vi "Stop Core.vi"(10 "final error code":i32 caption="最终错误代码", 11 "DAQ in":refnum<class "DAQ.lvclass"> caption="操作者输入") -> (3 "DAQ out":refnum<class "DAQ.lvclass"> caption="操作者输出")   [LabVIEW 2017, in "DAQ.lvlib" / "DAQ.lvclass"]
doc: "(<B>Filename</B>: Actor Framework.lvlib:Actor.lvclass:Stop Core.vi)\n\nDefines what the actor does before it stops. Use the <B>final error code</B> input to determine whether the actor shut down in response to an error.\n\nBy default, this method does nothing.子孙类重写该方法，定义出错时的操作，例如，关闭操作者核心方法初始的进程。"
uses:
  DAQ.lvclass
  DAQ.lvclass/DAQ.ctl
  <vilib>/ActorFramework/Actor/Actor.lvclass
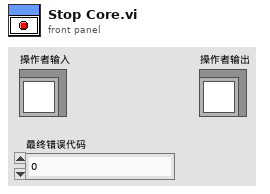
[diagram p1: front panel]
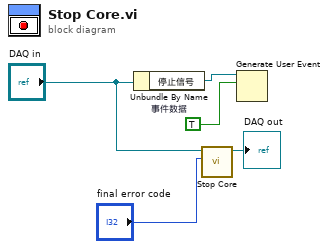
[diagram p0: block diagram]
diagram:
  w1 = TRUE  # 事件数据
  n1 = Unbundle By Name("DAQ in") -> ("停止信号"=w2:refnum<user-event>)
  n2 = call-parent "Stop Core.vi"("final error code"="final error code", "Actor in"="DAQ in") -> ("Actor out"=→"DAQ out":refnum<class "DAQ.lvclass">)  [unwired: 9 in]
  n3 = Generate User Event(user event=w2, event data cluster=w1) -> ()  [unwired: 2 in, 2 out]
